vi "Modbus Get Initial Gas Valve Setting.vi"(8 "error in (no error)":errorcluster, 9 "LDO Input":bool[](array[boolean]), 10 "FVIR Input":bool[](array[boolean]), 11 "Modbus Master in":refnum<class "Modbus Master.lvclass">) -> (0 "error out":errorcluster, 1 "LDO Output":bool[](array[boolean]), 2 "FVIR Output":bool[](array[boolean]), 3 "Modbus Master out":refnum<class "Modbus Master.lvclass">)   [LabVIEW 2020, in "Modbus.lvlib"]
uses:
  Modbus.lvlib
  <vilib>/NI/Modbus Library/API/Master/Modbus Master.lvclass
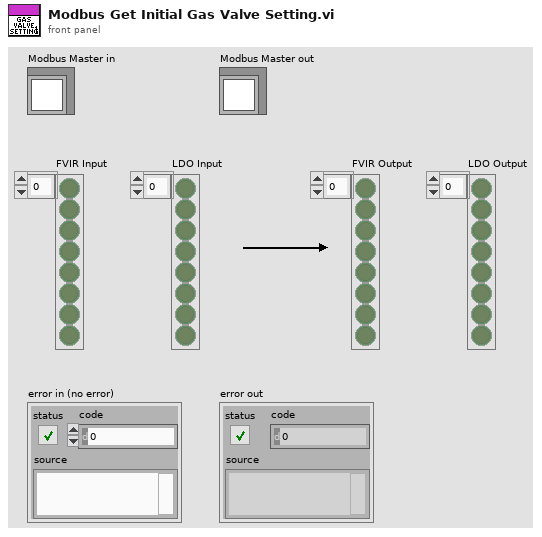
[diagram p1: front panel]
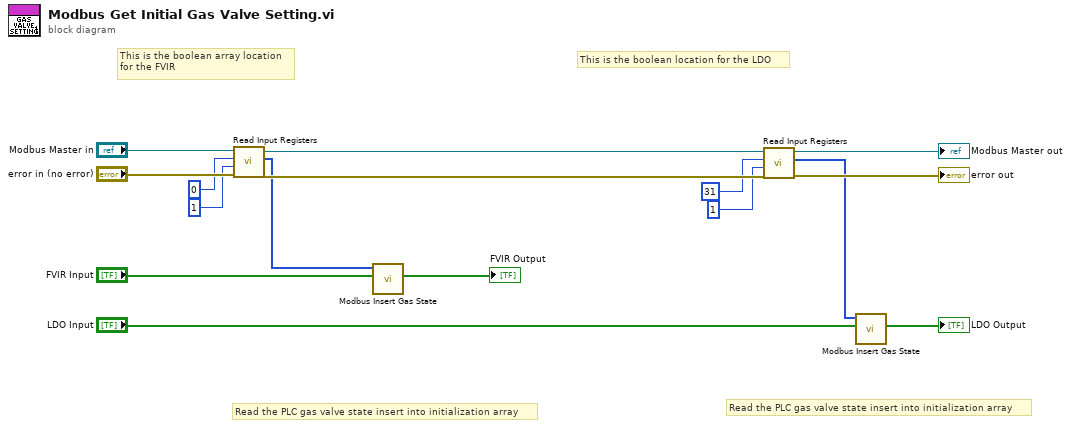
[diagram p0: block diagram]
diagram:
  # "This is the boolean location for the LDO"
  # "This is the boolean array location\nfor the FVIR"
  # "Read the PLC gas valve state insert into initialization array"
  # "Read the PLC gas valve state insert into initialization array"
  n1 = call-dynamic "Read Input Registers.vi"("error in"="error in (no error)", "number of inputs"=u16 1, "starting address"=u16 0, "Modbus master in"="Modbus Master in") -> ("error out"=w12:errorcluster, "register values"=w6:u16[], "Modbus master out"=w11:refnum<class "Modbus Master.lvclass">)  [unwired: 5 in]
  n2 = call "Modbus Insert Gas State.vi"("Array Input"="FVIR Input", "register values"=w6) -> ("Array Output"=→"FVIR Output":bool[])  [unwired: 8 in, 1 out]
  n3 = call-dynamic "Read Input Registers.vi"("error in"=w12, "number of inputs"=u16 1, "starting address"=u16 31, "Modbus master in"=w11) -> ("error out"=→"error out":errorcluster, "register values"=w3:u16[], "Modbus master out"=→"Modbus Master out":refnum<class "Modbus Master.lvclass">)  [unwired: 5 in]
  n4 = call "Modbus Insert Gas State.vi"("Array Input"="LDO Input", "register values"=w3) -> ("Array Output"=→"LDO Output":bool[])  [unwired: 8 in, 1 out]
